vi "GlobalTimingMode.vi"() -> ()   [LabVIEW 2010]
panel:
  in  "Timing Mode":u32
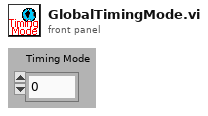
[diagram p1: front panel]
diagram:
